vi "Prime BSI Live Preview.vi"(0 "Notifier In":refnum<notifier>, 7 "Camera Ref":refnum<k24>, 11 "Error In":errorcluster, 13 "Image Ref":T1) -> (4 "Notifier Out":refnum<notifier>, 8 "Prime Cluster":T2, 15 "Error Out":errorcluster)   [LabVIEW 2020]
uses:
  C:/Users/Public/Documents/Photometrics/PMQI-LabViewSamples BETA/Examples/2020/Dependencies/PVCamNET.dll
  Public/Documents/Photometrics/PMQI-LabViewSamples BETA/Examples/2020/Dependencies/PVCamNET.dll
  Prime BSI Type Defs/Prime BSI Notifier Element.ctl
  Prime BSI Type Defs/Prime BSI Actions.ctl
  Prime BSI Type Defs/Prime BSI Parameters.ctl
  Prime BSI Type Defs/Prime BSI Parameter List.ctl
  Prime BSI Type Defs/Prime BSI ROI.ctl
  <vilib>/vision/Image Controls.llb/IMAQ Image.ctl
  Camera Controls/Camera IMAQ Key Info.ctl
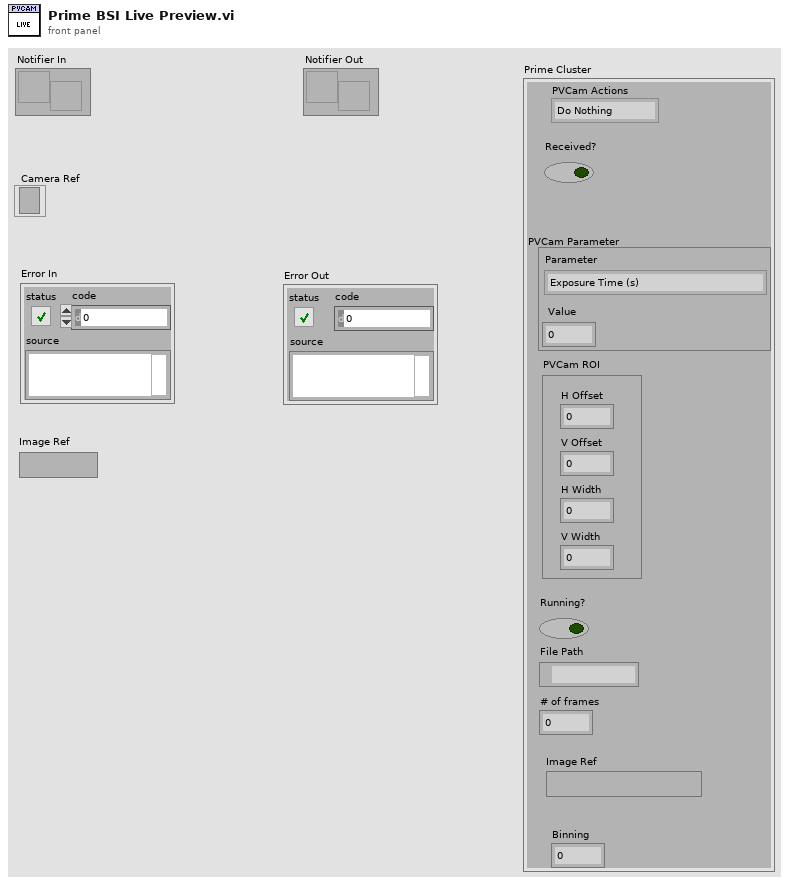
[diagram p1: front panel]
types:
  T1 = typedef "IMAQ Image.ctl" = refnum<image>
  T2 = typedef "Prime BSI Notifier Element.ctl" = cluster{"PVCam Actions":T3, "Received?":bool, "PVCam Parameter":T4, "PVCam ROI":T6, "Running?":bool, "File Path":path, "# of frames":u32, "Image Ref":T1, "Binning":i32}
  T3 = typedef "Prime BSI Actions.ctl" = enum16{"Do Nothing", "Preview", "Record", "Abort", "Record Settings", "Set Parameter", "Get Parameter", "Set ROI", "Get ROI", "Status", "Quit"}
  T4 = typedef "Prime BSI Parameters.ctl" = cluster{"Parameter":T5, "Value":dbl}
  T5 = typedef "Prime BSI Parameter List.ctl" = enum16{"Exposure Time (s)", "Binning"}
  T6 = typedef "Prime BSI ROI.ctl" = cluster{"H Offset":i32, "V Offset":i32, "H Width":i32, "V Width":i32}
  T7 = typedef "Camera IMAQ Key Info.ctl" = cluster{"Frame":u32, "Sensor Height":i32, "Sensor Width":i32, "ROI Height":i32, "ROI Width":i32, "ROI Enable?":bool, "Bit per Pixel":u8}
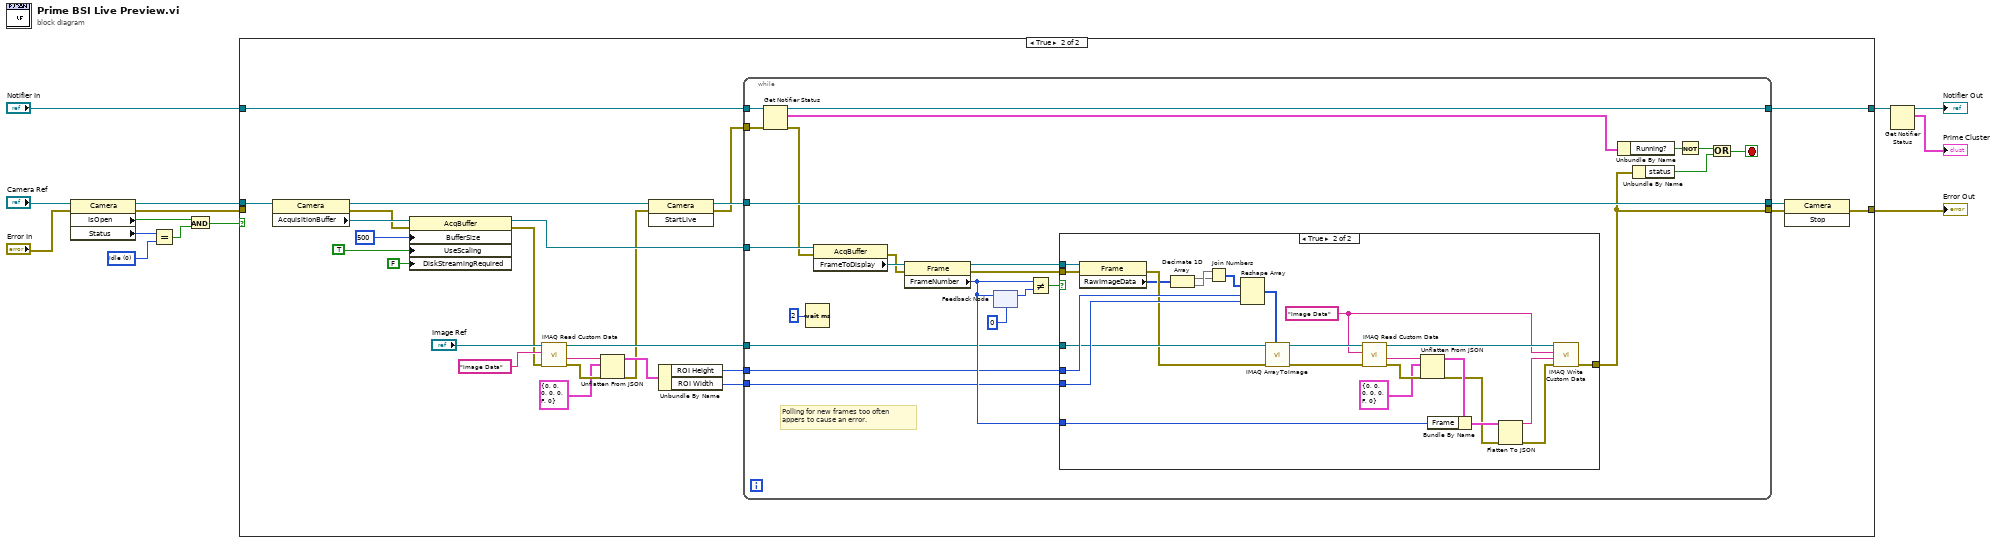
[diagram p0: block diagram]
diagram:
  w13 = 0 items=["Idle", "Capturing"] ("Status")
  n1 = property class="Camera"(reference="Camera Ref", error in="Error In") -> (reference out=w7:refnum<k24>, error out=w6:errorcluster, "IsOpen"=w12:bool, "Status"=w14:i32)
  n2 = Equal?(x=w14, y=w13) -> (x = y?=w11:bool)
  n3 = And(x=w12, y=w11) -> (x .and. y?=w8:bool)
  n4 = case shown="True" w8 {
    tunnel: w7 -> [_ w21]
    tunnel: w6 -> [w15 _]
    tunnel: "Notifier In" -> [w16 w40]
    tunnel: [w16 w36] -> w3
    tunnel: [w15 w35] -> w4
    frame False {
    }
    frame True {
      n5 = property class="Camera"(reference=w21) -> (reference out=w20:refnum<k24>, error out=w17:errorcluster, "AcquisitionBuffer"=w42:refnum<k24>)  [unwired: 1 in]
      n6 = property class="AcqBuffer"(reference=w42, error in=w17, "BufferSize"=u32 500, "UseScaling"=TRUE, "DiskStreamingRequired"=FALSE) -> (reference out=w34:refnum<k24>, error out=w27:errorcluster)
      n7 = call "IMAQ Read Custom Data"("error in (no error)"=w27, "Key"="Image Data", "Image"="Image Ref") -> ("error out"=w31:errorcluster, "Custom Data Out"=w32:string, "Image (duplicate)"=w24:T1)  [unwired: 6 in]
      n8 = Unflatten From JSON(JSON string=w32, type and defaults=T7 {"Frame"=0, "Sensor Height"=0, "Sensor Width"=0, "ROI Height"=0, "ROI Width"=0, "ROI Enable?"=FALSE, "Bit per Pixel"=0} ("Camera IMAQ Key Info"), error in (no error)=w31) -> (value=w28:T7, error out=w19:errorcluster)  [unwired: 4 in]
      n9 = invoke class="Camera" method="StartLive"(reference=w20, error in=w19) -> (reference out=w39:refnum<k24>, error out=w38:errorcluster)  [unwired: 1 in, 1 out]
      n10 = Unbundle By Name(w28) -> ("ROI Height"=w26:i32, "ROI Width"=w25:i32)
      n11 = while {
        tunnel: w40 -> [w66]
        tunnel: w39 -> [w58]
        tunnel: w38 -> [w64]
        tunnel: [w58] -> w37
        tunnel: [w59] -> w36
        tunnel: w34 -> [w57]
        tunnel: w26 -> [w49]
        tunnel: w25 -> [w48]
        tunnel: w24 -> [w50]
        tunnel: [w44] -> w23
        stop <- w62 stop-if-true
        # "Polling for new frames too often\nappers to cause an error."
        n12 = Get Notifier Status(notifier=w66, error in (no error)=w64) -> (notifier out=w59:refnum<notifier>, current notification=w60:T2, error out=w47:errorcluster)  [unwired: 2 out]
        n13 = Wait (ms)(milliseconds to wait=u32 2) -> ()  [unwired: 1 out]
        n14 = property class="AcqBuffer"(reference=w57, error in=w47) -> (error out=w46:errorcluster, "FrameToDisplay"=w56:refnum<k24>)  [unwired: 1 out]
        n15 = property class="Frame"(reference=w56, error in=w46) -> (reference out=w52:refnum<k24>, error out=w45:errorcluster, "FrameNumber"=w51:u32)
        n16 = feedback-in #1(w51) -> ()
        n17 = feedback #1(u32 0 ("FrameNumber")) -> (w54:u32)
        n18 = Not Equal?(x=w51, y=w54) -> (x != y?=w53:bool)
        n19 = case shown="True" w53 {
          tunnel: w52 -> [_ w92]
          tunnel: w51 -> [_ w83]
          tunnel: w50 -> [_ w89]
          tunnel: w49 -> [_ w91]
          tunnel: w48 -> [_ w90]
          tunnel: w45 -> [w67 w75]
          tunnel: [w67 w73] -> w44
          frame False {
          }
          frame True {
            w76 = "Image Data" ("Key")
            n20 = property class="Frame"(reference=w92, error in=w75) -> (error out=w74:errorcluster, "RawImageData"=w72:u8[])  [unwired: 1 out]
            n21 = Decimate 1D Array(w72) -> (w70:u8[], w71:u8[])
            n22 = Join Numbers(hi=w71, lo=w70) -> ((hi.lo)=w69:u16[])
            n23 = Reshape Array(w69, w91, w90) -> (w68:u16[][])
            n24 = call "IMAQ ArrayToImage"("Image Pixels (U16)"=w68, "error in (no error)"=w74, "Image"=w89) -> ("error out"=w84:errorcluster, "Image Out"=w85:T1)  [unwired: 7 in]
            n25 = call "IMAQ Read Custom Data"("error in (no error)"=w84, "Key"=w76, "Image"=w85) -> ("error out"=w87:errorcluster, "Custom Data Out"=w88:string, "Image (duplicate)"=w81:T1)  [unwired: 6 in]
            n26 = Unflatten From JSON(JSON string=w88, type and defaults=T7 {"Frame"=0, "Sensor Height"=0, "Sensor Width"=0, "ROI Height"=0, "ROI Width"=0, "ROI Enable?"=FALSE, "Bit per Pixel"=0} ("Camera IMAQ Key Info"), error in (no error)=w87) -> (value=w82:T7, error out=w79:errorcluster)  [unwired: 4 in]
            n27 = Bundle By Name(cluster=w82, "Frame"=w83) -> (w80:T7)
            n28 = Flatten To JSON(anything=w80, error in (no error)=w79) -> (JSON string=w78:string, 11:w77:errorcluster)  [unwired: 1 in]
            n29 = call "IMAQ Write Custom Data"("error in (no error)"=w77, "Custom Data In"=w78, "Key"=w76, "Image"=w81) -> ("error out"=w73:errorcluster)  [unwired: 6 in, 1 out]
          }
        }
        n30 = Unbundle By Name(w60) -> ("Running?"=w65:bool)
        n31 = Unbundle By Name(w44) -> ("status"=w61:bool)
        n32 = Not(x=w65) -> (.not. x?=w63:bool)
        n33 = Or(x=w63, y=w61) -> (x .or. y?=w62:bool)
      }
      n34 = invoke class="Camera" method="Stop"(reference=w37, error in=w23) -> (error out=w35:errorcluster)  [unwired: 1 in, 2 out]
    }
  }
  "Error Out" <- w4
  n35 = Get Notifier Status(notifier=w3) -> (notifier out=→"Notifier Out":refnum<notifier>, current notification=→"Prime Cluster":T2)  [unwired: 1 in, 3 out]
